vi "Check Variable Exist.vi"(8 "error in (no error)":errorcluster, 9 "Name":string, 10 "Variable Type":enum16{"Project", "Execution"}(ring), 11 "Project in":refnum<class "Project.lvclass">) -> (0 "error out":errorcluster, 1 "Exist":bool, 3 "Project out":refnum<class "Project.lvclass">)   [LabVIEW 2015, in "Project.lvclass"]
uses:
  Project.lvclass
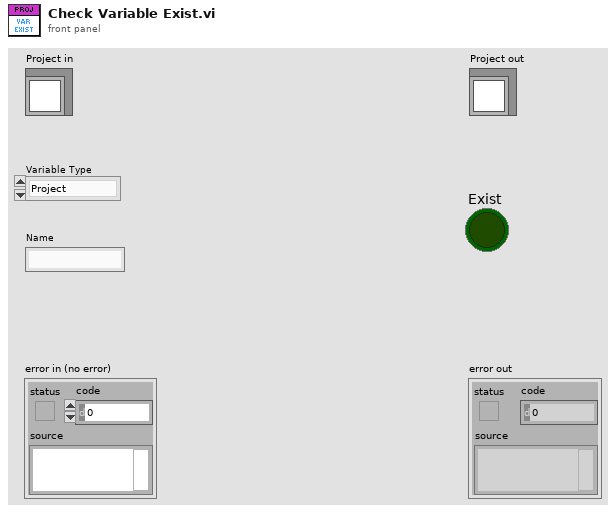
[diagram p1: front panel]
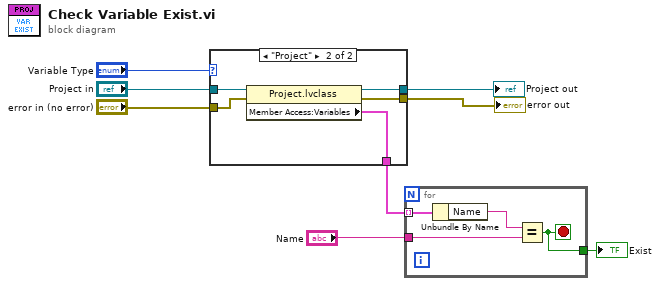
[diagram p0: block diagram]
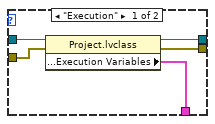
[diagram p2: hidden frame]
diagram:
  n1 = case shown="\"Project\"" "Variable Type" {
    tunnel: "Project in" -> [w13 w18]
    tunnel: [w12 w17] -> w8
    tunnel: [w11 w16] -> w6
    tunnel: [w10 w15] -> w4
    tunnel: "error in (no error)" -> [w9 w14]
    frame "Execution" {
      n2 = property class="Project.lvclass"(reference=w13, error in=w9) -> (reference out=w11:refnum<class "Project.lvclass">, error out=w10:errorcluster, "Member Access:Execution Variables"=w12:cluster{"Name":string, "Value":variant}[])
    }
    frame "Project" {
      n3 = property class="Project.lvclass"(reference=w18, error in=w14) -> (reference out=w16:refnum<class "Project.lvclass">, error out=w15:errorcluster, "Member Access:Variables"=w17:cluster{"Name":string, "Value":variant}[])
    }
  }
  "error out" <- w4
  "Project out" <- w6
  n4 = for {
    tunnel: w8 -> [w22] mode=indexing
    tunnel: "Name" -> [w20]
    tunnel: [w19] -> w1
    stop <- w19 stop-if-true
    n5 = Unbundle By Name(w22) -> ("Name"=w21:string)
    n6 = Equal?(x=w21, y=w20) -> (x = y?=w19:bool)
  }
  "Exist" <- w1
